vi "XY Graph Load Plot(s) from ASCII File.vi"(4 "Default X step (1)":dbl=1.0, 6 "Default X start (0)":dbl, 7 "Header Definitions":T2, 8 "error in (no error)":errorcluster, 9 "Delimiter (TAB)":string="\t", 10 "Abscissa Column? (T)":bool=TRUE, 11 "File Path":path) -> (0 "error out":errorcluster, 1 "Plot Scales Array":T1[](array[typedef]), 2 "Plot Name Array":string[](array[string]), 3 "Plot Array":cluster{"X Array":dbl[], "Y Array":dbl[]}[](array[cluster]))   [LabVIEW 2021, in "XY Graph Add-Ons.lvlib"]
uses:
  XY Graph Add-Ons.lvlib
  Files/ASCII File Header Definition.ctl
  XY Graph Plot Scale Labels.ctl
  Time/Time.lvlib
  Files/Files.lvlib
panel:
  out "Time (s)":dbl
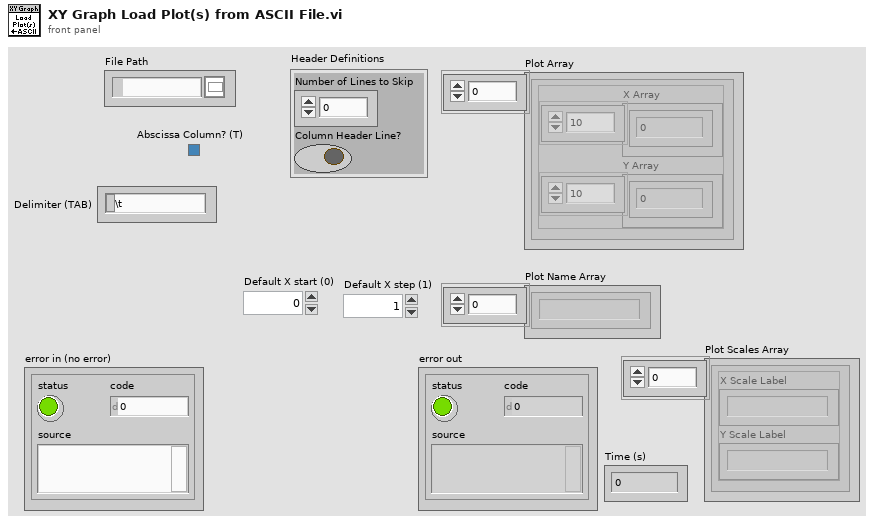
[diagram p1: front panel]
types:
  T1 = typedef "XY Graph Add-Ons.lvlib/XY Graph Plot Scale Labels.ctl" = cluster{"X Scale Label":string, "Y Scale Label":string}
  T2 = typedef "Files.lvlib/ASCII File Header Definition.ctl" = cluster{"Number of Lines to Skip":i32, "Column Header Line?":bool}
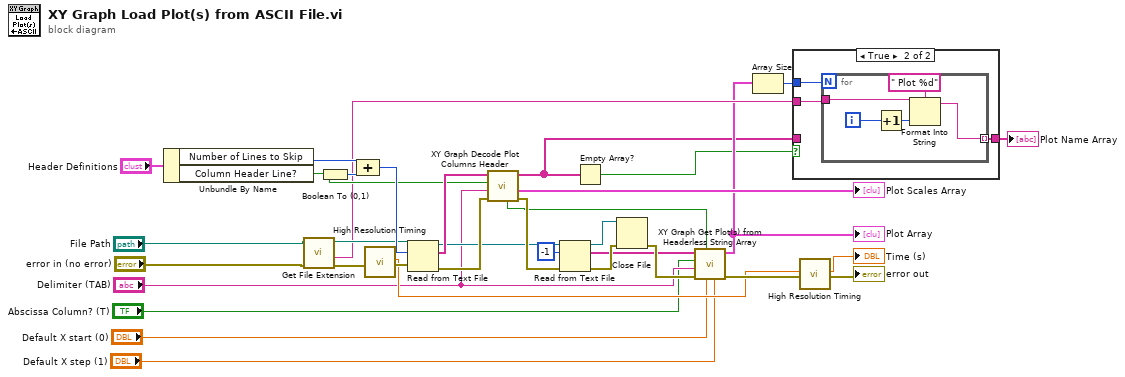
[diagram p0: block diagram]
diagram:
  n1 = Unbundle By Name("Header Definitions") -> ("Number of Lines to Skip"=w34:i32, "Column Header Line?"=w29:bool)
  n2 = call <vilib>:"Get File Extension.vi"("error in (no error)"="error in (no error)", "file"="File Path") -> ("error out"=w10:errorcluster, "filename without extension"=w9:string, "dup file"=w11:path)  [unwired: 5 in, 2 out]
  n3 = Boolean To (0,1)(Boolean=w29) -> (0, 1=w33:i16)
  n4 = Compound Arithmetic op=ADD(w34, w33) -> (w32:i32)
  n5 = call "High Resolution Timing.vi"("Error In"=w10) -> ("elapsed (relative) seconds"=w24:dbl, "Error Out"=w27:errorcluster)  [unwired: 16 in, 1 out]
  n6 = Read from Text File(file (use dialog)=w11, count=w32, error in=w27) -> (refnum out=w19:refnum<file>, text=w31:string[], error out=w30:errorcluster)  [unwired: 1 in, 1 out]
  n7 = call "XY Graph Decode Plot Columns Header.vi"("Error In"=w30, "Delimiter"="Delimiter (TAB)", "Column Header Line? (F)"=w29, "Header String Array"=w31) -> ("Error Out"=w22:errorcluster, "Plot Scales Array"=→"Plot Scales Array":T1[], "Plot Name Array"=w4:string[], "Alternating Axes?"=w14:bool)  [unwired: 4 in]
  n8 = Read from Text File(file (use dialog)=w19, count=-1, error in=w22) -> (refnum out=w20:refnum<file>, text=w15:string[], error out=w18:errorcluster)  [unwired: 1 in, 1 out]
  n9 = Empty Array?(array=w4) -> (empty?=w6:bool)
  n10 = Close File(refnum=w20, error in=w18) -> (error out=w17:errorcluster)  [unwired: 1 out]
  n11 = call "XY Graph Get Plot(s) from Headerless String Array.vi"("Default X step (1)"="Default X step (1)", "Default X start (0)"="Default X start (0)", "Alternating Axes?"=w14, "error in (no error)"=w17, "Delimiter"="Delimiter (TAB)", "Abscissa Column? (T)"="Abscissa Column? (T)", "Text Lines"=w15) -> ("error out"=w26:errorcluster, "Plot Array"=w7:cluster{"Array":dbl[], "Array":dbl[]}[])  [unwired: 3 in]
  "Plot Array" <- w7
  n12 = Array Size(array=w7) -> (size(s)=w5:i32)
  n13 = case shown="True" w6 {
    tunnel: w9 -> [_ w39]
    tunnel: [w36 w38] -> w8
    tunnel: w5 -> [_ w37]
    tunnel: w4 -> [w36 _]
    frame False {
    }
    frame True {
      n14 = for {
        N: w37 -> [_]
        tunnel: w39 -> [w44]
        tunnel: [w40] -> w38 mode=indexing
        i -> [w42]
        n15 = Increment(x=w42) -> (x+1=w41:i32)
        n16 = Format Into String(format string=" Plot %d", initial string=w44, w41) -> (resulting string=w40:string)  [unwired: 1 in, 1 out]
      }
    }
  }
  "Plot Name Array" <- w8
  n17 = call "High Resolution Timing.vi"("relative seconds (NaN)"=w24, "Error In"=w26) -> ("elapsed (relative) seconds"=→"Time (s)":dbl, "Error Out"=→"error out":errorcluster)  [unwired: 15 in, 1 out]
